vi "ChangeOneRecordTo2DListCtrl.vi"(9 "all data?":bool, 10 "배열":string[](array[string]), 11 "testcaselist in":refnum<vi>) -> (3 "testcaselist out":refnum<vi>)   [LabVIEW 2018, in "Library-Ctrl.lvlib"]
uses:
  Library-Ctrl.lvlib
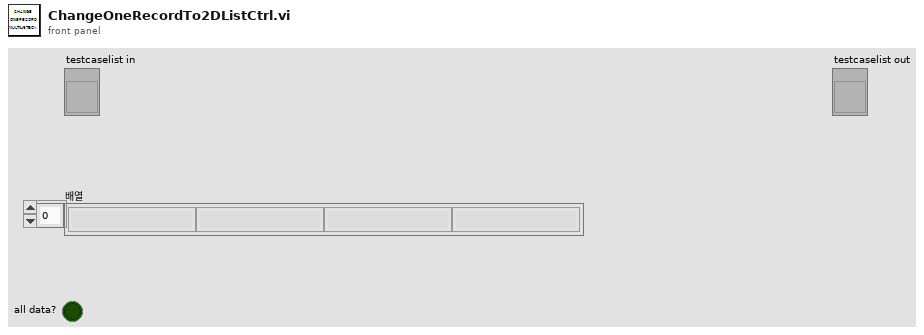
[diagram p1: front panel]
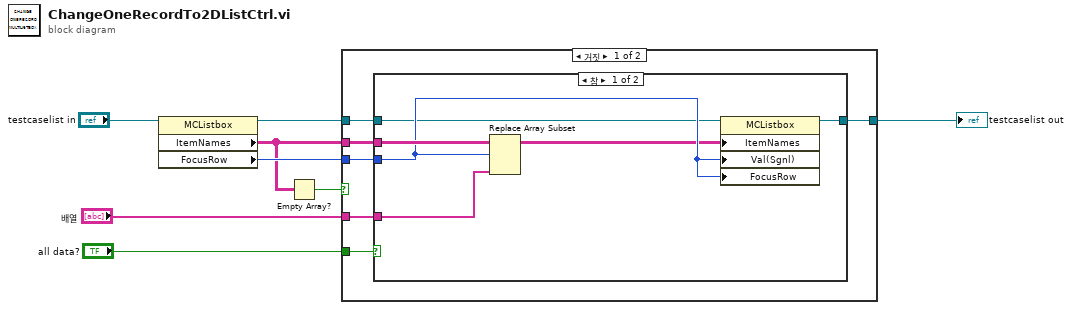
[diagram p0: block diagram]
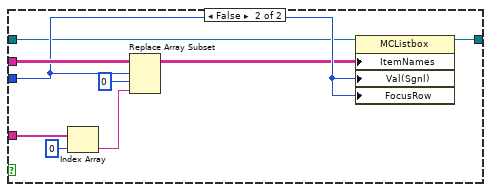
[diagram p2: hidden frame]
diagram:
  n1 = property class="MCListbox"(reference="testcaselist in") -> (reference out=w6:refnum<vi>, "ItemNames"=w4:string[][], "FocusRow"=w5:i32)  [unwired: 1 in, 1 out]
  n2 = Empty Array?(array=w4) -> (empty?=w7:bool)
  n3 = case shown="거짓" w7 {
    tunnel: w6 -> [w11 w30]
    tunnel: w5 -> [w12 _]
    tunnel: w4 -> [w14 _]
    tunnel: "배열" -> [w10 _]
    tunnel: [w13 w30] -> w3
    tunnel: "all data?" -> [w9 _]
    frame False {
      n4 = case shown="참" w9 {
        tunnel: w14 -> [w20 w29]
        tunnel: [w19 w28] -> w13
        tunnel: w12 -> [w18 w27]
        tunnel: w11 -> [w16 w25]
        tunnel: w10 -> [w15 w24]
        frame True {
          n5 = Replace Array Subset(array=w20, new element=w15, index (row)=w18) -> (w17:string[][])  [unwired: 1 in]
          n6 = property class="MCListbox"(reference=w16, "ItemNames"=w17, "Val(Sgnl)"=w18, "FocusRow"=w18) -> (reference out=w19:refnum<vi>)  [unwired: 1 in, 1 out]
        }
        frame False {
          n7 = Index Array(array=w24, index=0 ("인덱스")) -> (element=w21:string)
          n8 = Replace Array Subset(array=w29, new element=w21, index (row)=w27, index (col)=0 ("비활성화된 인덱스 (열)")) -> (w26:string[][])
          n9 = property class="MCListbox"(reference=w25, "ItemNames"=w26, "Val(Sgnl)"=w27, "FocusRow"=w27) -> (reference out=w28:refnum<vi>)  [unwired: 1 in, 1 out]
        }
      }
    }
    frame True {
    }
  }
  "testcaselist out" <- w3
